vi "TCL Get Datalog Records.vi"(2 "error in (no error)":errorcluster, 3 "event file":path) -> (0 "error out":errorcluster, 1 "records":string[][](array[string]))   [LabVIEW 2010]
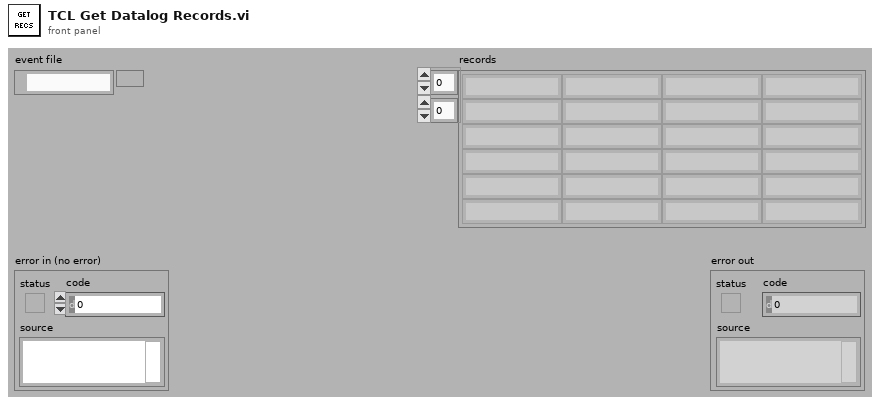
[diagram p1: front panel]
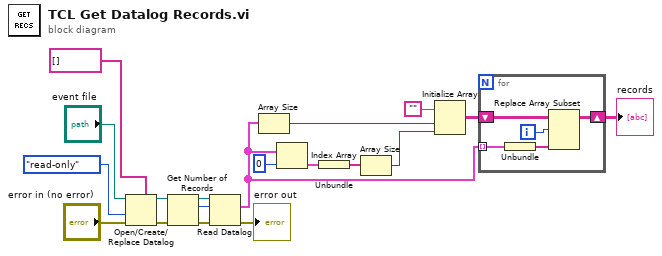
[diagram p0: block diagram]
diagram:
  n1 = Open/Create/Replace Datalog(5:string[] [], 8:"error in (no error)", 9:enum16{"read/write", "read-only", "write-only"}."read-only" ("access (0:read/write)"), 11:"event file") -> (0:w15:errorcluster, 3:w14:refnum<k1>)  [unwired: 2 in, 1 out]
  n2 = Get Number of Records(4:w15, 7:w14) -> (0:w13:errorcluster, 2:w12:i64, 3:w11:refnum<k1>)
  n3 = Read Datalog(4:w13, 6:w12, 7:w11) -> (0:→"error out":errorcluster, 2:w5:cluster{string[]}[])  [unwired: 1 out]
  n4 = Array Size(array=w5) -> (size(s)=w6:i32)
  n5 = Index Array(array=w5, index=0) -> (element=w3:cluster{string[]})
  n6 = Unbundle(w3) -> (w2:string[])
  n7 = Array Size(array=w2) -> (size(s)=w1:i32)
  n8 = Initialize Array("", w6, w1) -> (w8:string[][])
  n9 = for {
    tunnel: w5 -> [w23] mode=indexing
    shift-right: [w22] -> w9
    shift-left: w8 -> [w24]
    i -> [w20]
    n10 = Unbundle(w23) -> (w21:string[])
    n11 = Replace Array Subset(array=w24, new element=w21, index (row)=w20) -> (w22:string[][])  [unwired: 1 in]
  }
  "records" <- w9
